vi "clear_sailing_points.vi"(1 "Waypoints queue":refnum<queue>) -> (0 "Waypoints queue 2":refnum<queue>)   [LabVIEW 2013]
uses:
  Logic/Classes/Waypoint/Waypoint.lvclass
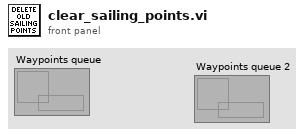
[diagram p1: front panel]
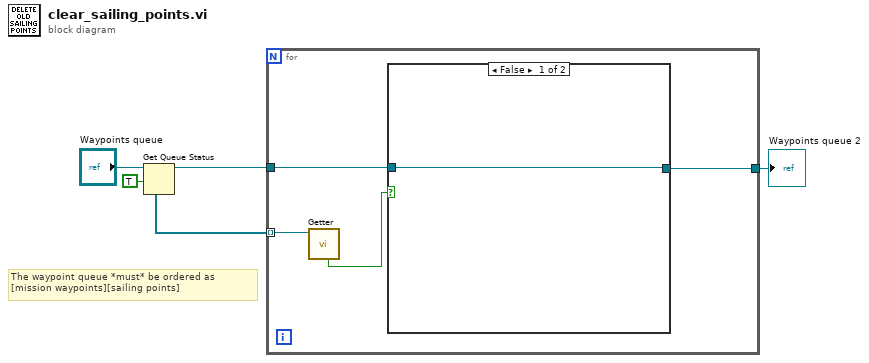
[diagram p0: block diagram]
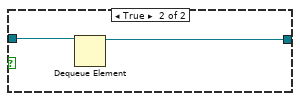
[diagram p2: hidden frame]
diagram:
  # "The waypoint queue *must* be ordered as [mission waypoints][sailing points]"
  n1 = Get Queue Status(queue="Waypoints queue", return elements? (F)=TRUE) -> (queue out=w4:refnum<queue>, elements=w2:refnum<class "Waypoint.lvclass">[])  [unwired: 1 in, 6 out]
  n2 = for {
    tunnel: w4 -> [w9]
    tunnel: w2 -> [w8] mode=indexing
    tunnel: [w6] -> w1
    n3 = call "Getter.vi"("Waypoint In"=w8) -> ("Sailing Point?"=w7:bool)  [unwired: 5 in, 5 out]
    n4 = case shown="False" w7 {
      tunnel: w9 -> [w10 w12]
      tunnel: [w10 w11] -> w6
      frame False {
      }
      frame True {
        n5 = Dequeue Element(queue=w12) -> (queue out=w11:refnum<queue>)  [unwired: 2 in, 3 out]
      }
    }
  }
  "Waypoints queue 2" <- w1
